vi "Start FGEN.vi"(8 "error in (no error)":errorcluster, 11 "Data In":T1 {"Toggle Channels"."Initial State" items=["High"=101, "Low"=102]; "Sample Rate" format="%.2p"}) -> (0 "error out":errorcluster, 3 "Data Out":T1 {"Toggle Channels"."Initial State" items=["High"=101, "Low"=102]; "Sample Rate" format="%.2p"})   [LabVIEW 2021]
uses:
  Controls/Data.ctl
  Controls/Script Trigger Routing.ctl
  Controls/Toggle Channel.ctl
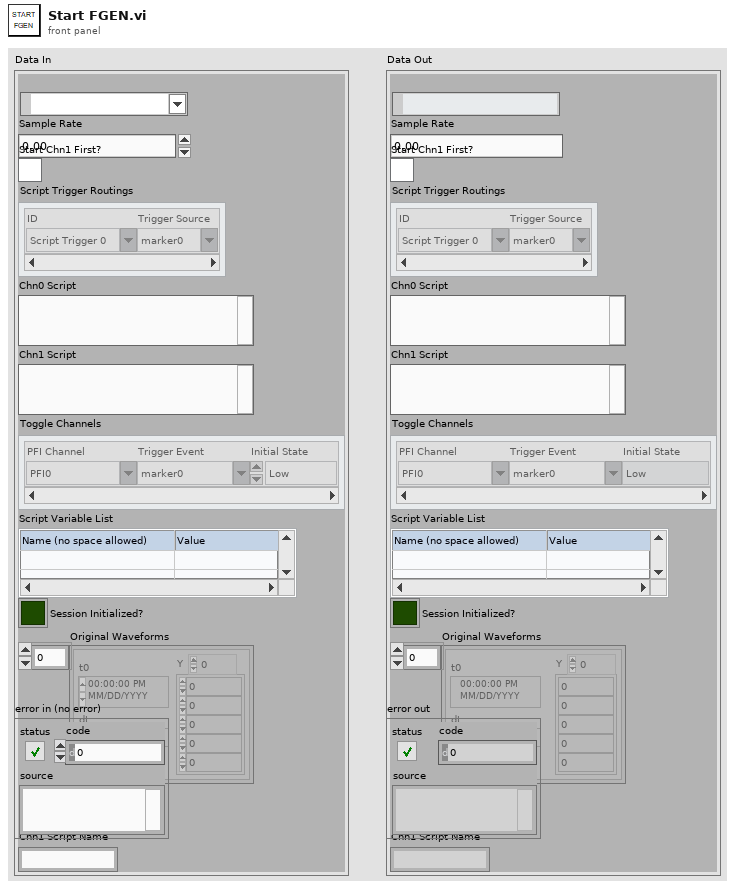
[diagram p1: front panel]
types:
  T1 = typedef "Data.ctl" = cluster{"FGEN Resource Name":refnum<k15>, "Sample Rate":dbl, "Start Chn1 First?":bool, "Script Trigger Routings":T2[], "Chn0 Script":string, "Chn1 Script":string, "Toggle Channels":T3[], "Script Variable List":string[][], "Session Initialized?":bool, "Original Waveforms":waveform(dbl)[], "Chn0 Script Name":string, "Chn1 Script Name":string}
  T2 = typedef "Script Trigger Routing.ctl" = cluster{"ID":string, "Trigger Source":string}
  T3 = typedef "Toggle Channel.ctl" = cluster{"PFI Channel":string, "Trigger Event":string, "Initial State":u16}
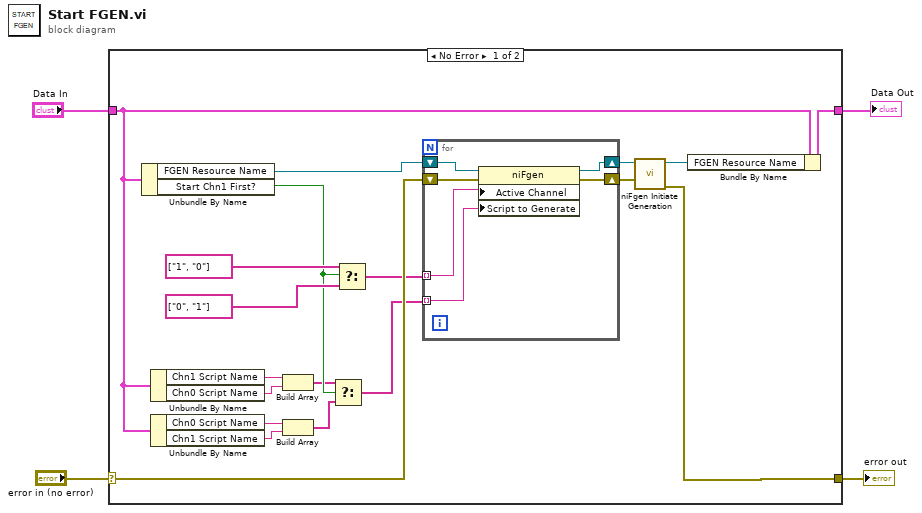
[diagram p0: block diagram]
diagram:
  n1 = case shown="No Error" "error in (no error)" {
    selector: "error in (no error)" -> [w21 w31]
    tunnel: "Data In" -> [w18 w30]
    tunnel: [w8 w30] -> w3
    tunnel: [w7 w31] -> w1
    frame No Error {
      n2 = Unbundle By Name(w18) -> ("FGEN Resource Name"=w23:refnum<k15>, "Start Chn1 First?"=w13:bool)
      n3 = Unbundle By Name(w18) -> ("Chn1 Script Name"=w15:string, "Chn0 Script Name"=w14:string)
      n4 = Unbundle By Name(w18) -> ("Chn0 Script Name"=w17:string, "Chn1 Script Name"=w16:string)
      n5 = Build Array(w15, w14) -> (w11:string[])
      n6 = Build Array(w17, w16) -> (w12:string[])
      n7 = Select(t=w11, s=w13, f=w12) -> (s? t:f=w10:string[])
      n8 = Select(t=string[] ["1", "0"], s=w13, f=string[] ["0", "1"]) -> (s? t:f=w9:string[])
      n9 = for {
        shift-right: [w24] -> w22
        shift-left: w21 -> [w28]
        tunnel: w10 -> [w26] mode=indexing
        tunnel: w9 -> [w27] mode=indexing
        shift-right: [w25] -> w6
        shift-left: w23 -> [w29]
        n10 = property class="niFgen"(reference=w29, error in=w28, "Active Channel"=w27, "Script to Generate"=w26) -> (reference out=w25:refnum<k15>, error out=w24:errorcluster)
      }
      n11 = call <instrlib>:"niFgen Initiate Generation.vi"("error in (no error)"=w22, "Instrument Handle"=w6) -> ("error out"=w7:errorcluster, "Instrument Handle Out"=w5:refnum<k15>)  [unwired: 8 in]
      n12 = Bundle By Name(cluster=w18, "FGEN Resource Name"=w5) -> (w8:T1)
    }
    frame Error {
    }
  }
  "Data Out" <- w3
  "error out" <- w1
